vi "点位模式.vi"() -> ()   [LabVIEW 2020]
uses:
  VIs/gts.lvlib
  VI1s/gts1.lvlib
panel:
  in  "Tab Control":enum32{"Page 1", "Page 2"}(tab)
  in  "Jog运动":bool
  in  "pPrm 3":cluster{"acc":dbl, "dec":dbl, "smooth":dbl}={"acc"=1.0, "dec"=1.0, "smooth"=0.0}
  out "PrfJog return":i16
  in  "vel 2":dbl=30.0
  out "setPrm return":i16
  out "setVel return":i16
  out "Update return":i16
  out "clrsts return":i16
  in  "清除状态":bool
  out "stage 3":i16
  out "comparestop return":i16[](array[numeric])
  out "比较2return":i16[](array[numeric])
  out "比较1return":i16[](array[numeric])
  out "comparestart return":i16[](array[numeric])
  in  "pPrm 4":T1={"encx"=1, "ency"=2, "source"=0, "outputType"=0, "startLevel"=1, "time"=20000, "maxerr"=20, "threshold"=0}
  out "布尔数组":bool[](array[boolean])
  out "pSts 2":i32
  out "error":i16
  out "pStatus out":i16
  out "pValue out 2":i32
  out "function return 7":i16
  out "function return 6":i16
  in  "pBuf1":i32[](array[numeric])
  in  "一维位置比较":bool
  out "添加的数组":i16[](array[numeric])
  in  "pCrdPrm 2":T2={"dimension"=3, "profile[0]"=1, "profile[1]"=2, "profile[2]"=3, "profile[3]"=0, "profile[4]"=0, "profile[5]"=0, "profile[6]"=0, "profile[7]"=0, "@dummy control@"=0, "@dummy control@"=0, "@dummy control@"=0, "@dummy control@"=0, "@dummy control@"=0, "@dummy control@"=0, "synVelMax"=10.0, "synAccMax"=1.0, "evenTime"=10, "setOriginFlag"=0, "originPos[0]"=0, "originPos[1]"=0, "originPos[2]"=0, "originPos[3]"=0, "originPos[4]"=0, "originPos[5]"=0, "originPos[6]"=0, "originPos[7]"=0}
  in  "三轴直线插补":bool
  out "x = y?":bool
  out "stage 2":i16
  out "stage":i16
  out "close return":i16
  in  "关卡":bool
  in  "启动位置比较":bool
  in  "停止位置比较":bool
  in  "pBuf":cluster{"px":i32, "py":i32}[](array[cluster])=[{"px"=0, "py"=5000}, {"px"=0, "py"=8000}, {"px"=0, "py"=10000}, {"px"=0, "py"=15000}, {"px"=0, "py"=18000}, {"px"=0, "py"=20000}]
  in  "pPrm 2":T1={"encx"=1, "ency"=1, "source"=0, "outputType"=0, "startLevel"=1, "time"=20000, "maxerr"=20, "threshold"=0}
  in  "位置比较":bool
  in  "mdl":i16
  out "function return 3":i16
  in  "value":u16
  in  "index":i16
  in  "SetDo":bool
  out "function return 2":i16
  in  "路径 2":path
  out "function return":i16
  in  "pDllName":string
  in  "初始化扩展模块":bool
  out "homezero return 3":i16
  out "gohome return 3":i16
  out "get home prm return 3":i16
  in  "插补10000段":bool
  out "pSpace out":i32
  out "捕获次数":i32
  out "pValue out":i32
  out "追踪次数":i32
  in  "自动测试":bool
  in  "pEvent":T3={"loop"=1, "type"=30000, "index"=1, "id"=1, "condition"=3, "@dummy control@"=0, "@dummy control@"=0, "@dummy control@"=0, "@dummy control@"=0, "value"=50000.0}
  in  "pTaskData":cluster{"mask":i16, "option":i16}={"mask"=1, "option"=0}
  in  "主轴":i16=1
  in  "从轴":i16=2
  in  "单次测试":bool
  out "捕获数组":i32[](array[numeric])
  in  "打开home捕获":bool
  in  "pLookAheadBuf":T4(array[cluster])
  in  "数据路径":path=path "C:/Users/Admin/Desktop/固高资料/watch/Crd_data.txt"
  in  "轴号":T5(ring)=enum."2"
  out "闭环返回值":i16[](array[numeric])
  in  "闭环PID参数":T6={"kp"=2.0, "ki"=0.0, "kd"=0.0, "kvff"=0.0, "kaff"=0.0, "integralLimit"=0, "derivativeLimit"=0, "limit"=32767}
  in  "闭环控制":bool
  out "updatemotion return":i16
  in  "更新运动":bool
  out "zero return":i16
  in  "清零":bool
  out "CrdStart return":i16
  out "crddata return":i16
  out "Lnxy return":i16
  out "setCrd return":i16
  out "lookahead":i16
  in  "pCrdPrm":T2={"dimension"=2, "profile[0]"=1, "profile[1]"=2, "profile[2]"=0, "profile[3]"=0, "profile[4]"=0, "profile[5]"=0, "profile[6]"=0, "profile[7]"=0, "@dummy control@"=0, "@dummy control@"=0, "@dummy control@"=0, "@dummy control@"=0, "@dummy control@"=0, "@dummy control@"=0, "synVelMax"=10.0, "synAccMax"=1.0, "evenTime"=10, "setOriginFlag"=0, "originPos[0]"=0, "originPos[1]"=0, "originPos[2]"=0, "originPos[3]"=0, "originPos[4]"=0, "originPos[5]"=0, "originPos[6]"=0, "originPos[7]"=0}
  in  "前瞻":bool
  in  "插补运动":bool
  out "实际速度":dbl[](array[numeric])=[0.0, 0.0, 0.0, 0.0, 0.0, 0.0, 0.0, 1.0]
  out "encvel return":i16=-5
  out "实际位置":dbl[](array[numeric])=[0.0, 0.0, 0.0, 0.0, 0.0, 0.0, 0.0, 1.0]
  out "encpos return":i16=-5
  out "规划位置":dbl[](array[numeric])=[0.0, 0.0, 0.0, 0.0, 0.0, 0.0, 0.0, 1.0]
  out "prfpos return":i16=-5
  out "规划速度":dbl[](array[numeric])=[0.0, 0.0, 0.0, 0.0, 0.0, 0.0, 0.0, 1.0]
  out "prfvel return":i16=-5
  out "homezero return":i16
  out "gethomests return":i16
  out "pHomeStatus out":T7={"run"=0, "stage"=100, "error"=0, "pad1"=0, "capturePos"=-1, "targetPos"=-1}
  out "gohome return":i16
  out "get home prm return":i16
  in  "pHomePrm":T8={"mode"=11, "moveDir"=1, "indexDir"=1, "edge"=0, "triggerIndex"=-1, "pad1[0]"=0, "pad1[1]"=0, "pad1[2]"=0, "velHigh"=100.0, "velLow"=3.0, "acc"=1.0, "dec"=1.0, "smoothTime"=20, "pad2[0]"=0, "pad2[1]"=1, "pad2[2]"=0, "homeOffset"=0, "searchHomeDistance"=0, "searchIndexDistance"=0, "escapeStep"=2000, "pad3[0]"=0, "pad3[1]"=0}
  out "JogStop return":i16
  out "getPrm return":i16
  in  "回原点":bool
  out "reset return":i16
  out "Axisoff return":i16
  out "stopreturn":i16
  out "updatereturn":i16
  out "pos return":i16
  out "vel return":i16
  in  "vel":dbl=30.0
  in  "pos":i32=50000
  out "set prmreturn":i16
  out "get prm return":i16
  in  "pPrm":T9={"acc"=1.0, "dec"=1.0, "velStart"=0.0, "smoothTime"=20}
  out "set trap return":i16
  out "Axison return":i16
  out "clrsts return":i16
  out "config return":i16
  in  "路径":path=path "C:/Users/Admin/Desktop/GTS800.cfg"
  out "open return":i16
  in  "关伺服":bool
  in  "停止":bool
  in  "点位运动":bool
  in  "开伺服":bool
  in  "开卡":bool
  # "位置速度显示"
  # "函数返回值"
  # "点位运动参数"
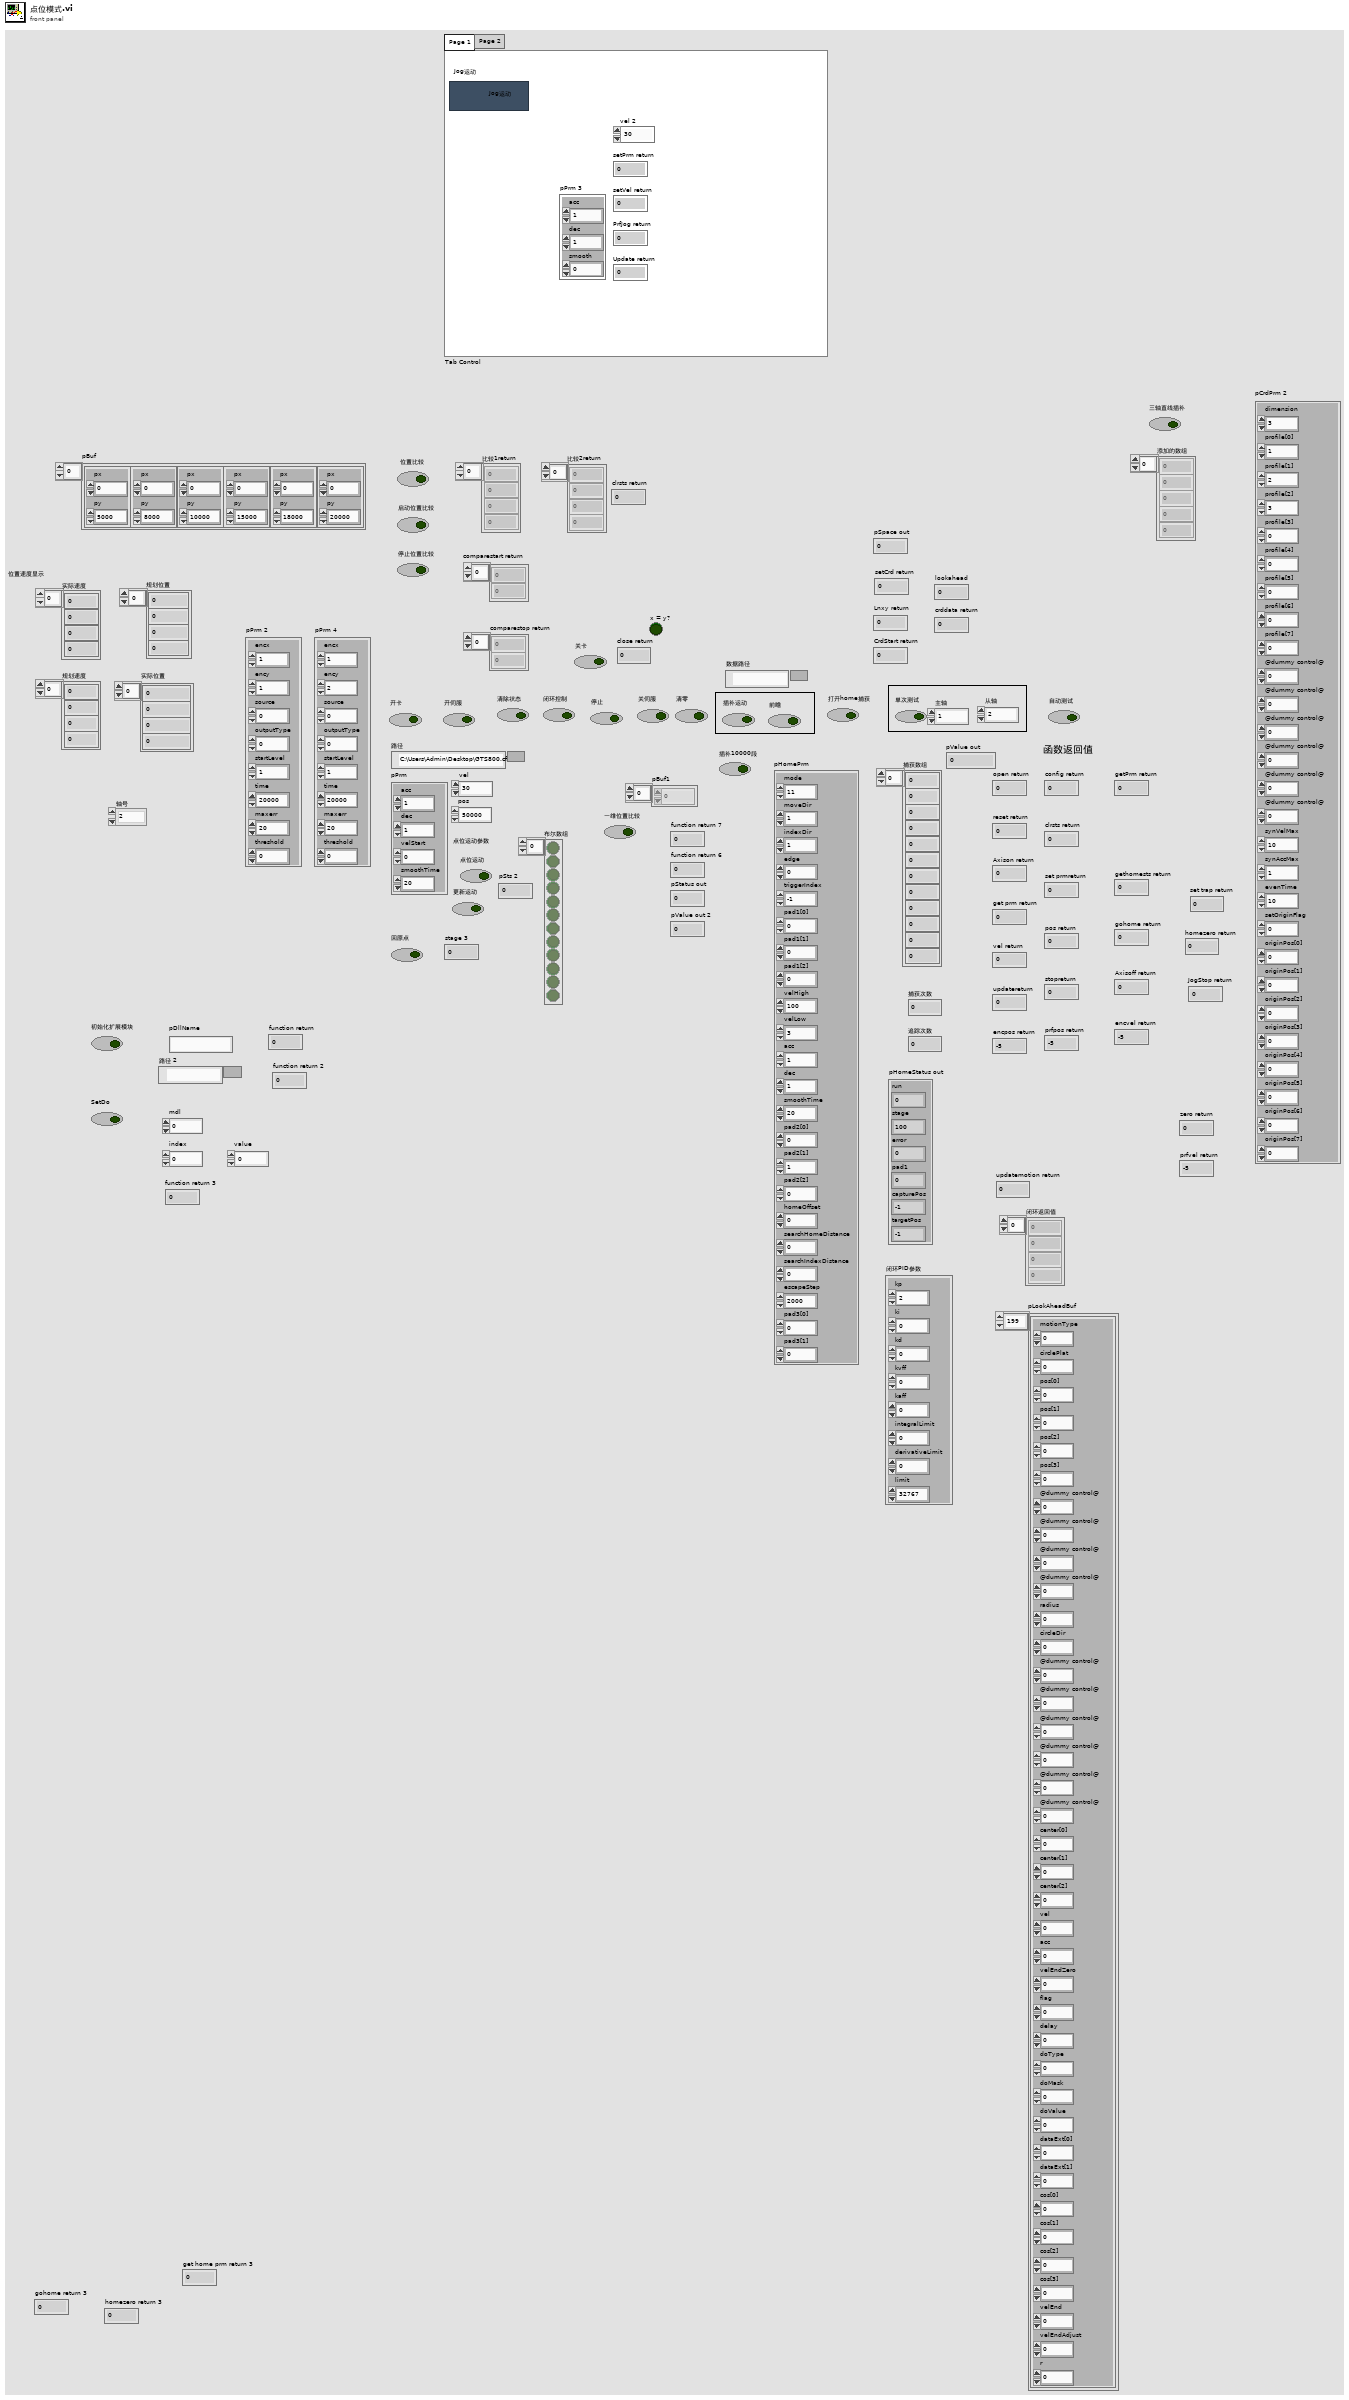
[diagram p1: front panel]
types:
  T1 = cluster{"encx":i16, "ency":i16, "source":i16, "outputType":i16, "startLevel":i16, "time":i16, "maxerr":i16, "threshold":i16}
  T2 = cluster{"dimension":i16, "profile[0]":i16, "profile[1]":i16, "profile[2]":i16, "profile[3]":i16, "profile[4]":i16, "profile[5]":i16, "profile[6]":i16, "profile[7]":i16, "@dummy control@":i8, "@dummy control@":i8, "@dummy control@":i8, "@dummy control@":i8, "@dummy control@":i8, "@dummy control@":i8, "synVelMax":dbl, "synAccMax":dbl, "evenTime":i16, "setOriginFlag":i16, "originPos[0]":i32, "originPos[1]":i32, "originPos[2]":i32, "originPos[3]":i32, "originPos[4]":i32, "originPos[5]":i32, "originPos[6]":i32, "originPos[7]":i32}
  T3 = cluster{"loop":u32, "type":u16, "index":u16, "id":u16, "condition":u16, "@dummy control@":i8, "@dummy control@":i8, "@dummy control@":i8, "@dummy control@":i8, "value":dbl}
  T4 = cluster{"motionType":i16, "circlePlat":i16, "pos[0]":i32, "pos[1]":i32, "pos[2]":i32, "pos[3]":i32, "@dummy control@":i8, "@dummy control@":i8, "@dummy control@":i8, "@dummy control@":i8, "radius":dbl, "circleDir":i16, "@dummy control@":i8, "@dummy control@":i8, "@dummy control@":i8, "@dummy control@":i8, "@dummy control@":i8, "@dummy control@":i8, "center[0]":dbl, "center[1]":dbl, "center[2]":dbl, "vel":dbl, "acc":dbl, "velEndZero":i16, "flag":i16, "delay":u16, "doType":i16, "doMask":u16, "doValue":u16, "dataExt[0]":u16, "dataExt[1]":u16, "cos[0]":dbl, "cos[1]":dbl, "cos[2]":dbl, "cos[3]":dbl, "velEnd":dbl, "velEndAdjust":dbl, "r":dbl}[]
  T5 = enum16{"none", "1", "2", "3", "4", "5", "6", "7", "8"}
  T6 = cluster{"kp":dbl, "ki":dbl, "kd":dbl, "kvff":dbl, "kaff":dbl, "integralLimit":i32, "derivativeLimit":i32, "limit":i16}
  T7 = cluster{"run":i16, "stage":i16, "error":i16, "pad1":i16, "capturePos":i32, "targetPos":i32}
  T8 = cluster{"mode":i16, "moveDir":i16, "indexDir":i16, "edge":i16, "triggerIndex":i16, "pad1[0]":i16, "pad1[1]":i16, "pad1[2]":i16, "velHigh":dbl, "velLow":dbl, "acc":dbl, "dec":dbl, "smoothTime":i16, "pad2[0]":i16, "pad2[1]":i16, "pad2[2]":i16, "homeOffset":i32, "searchHomeDistance":i32, "searchIndexDistance":i32, "escapeStep":i32, "pad3[0]":i32, "pad3[1]":i32}
  T9 = cluster{"acc":dbl, "dec":dbl, "velStart":dbl, "smoothTime":i16}
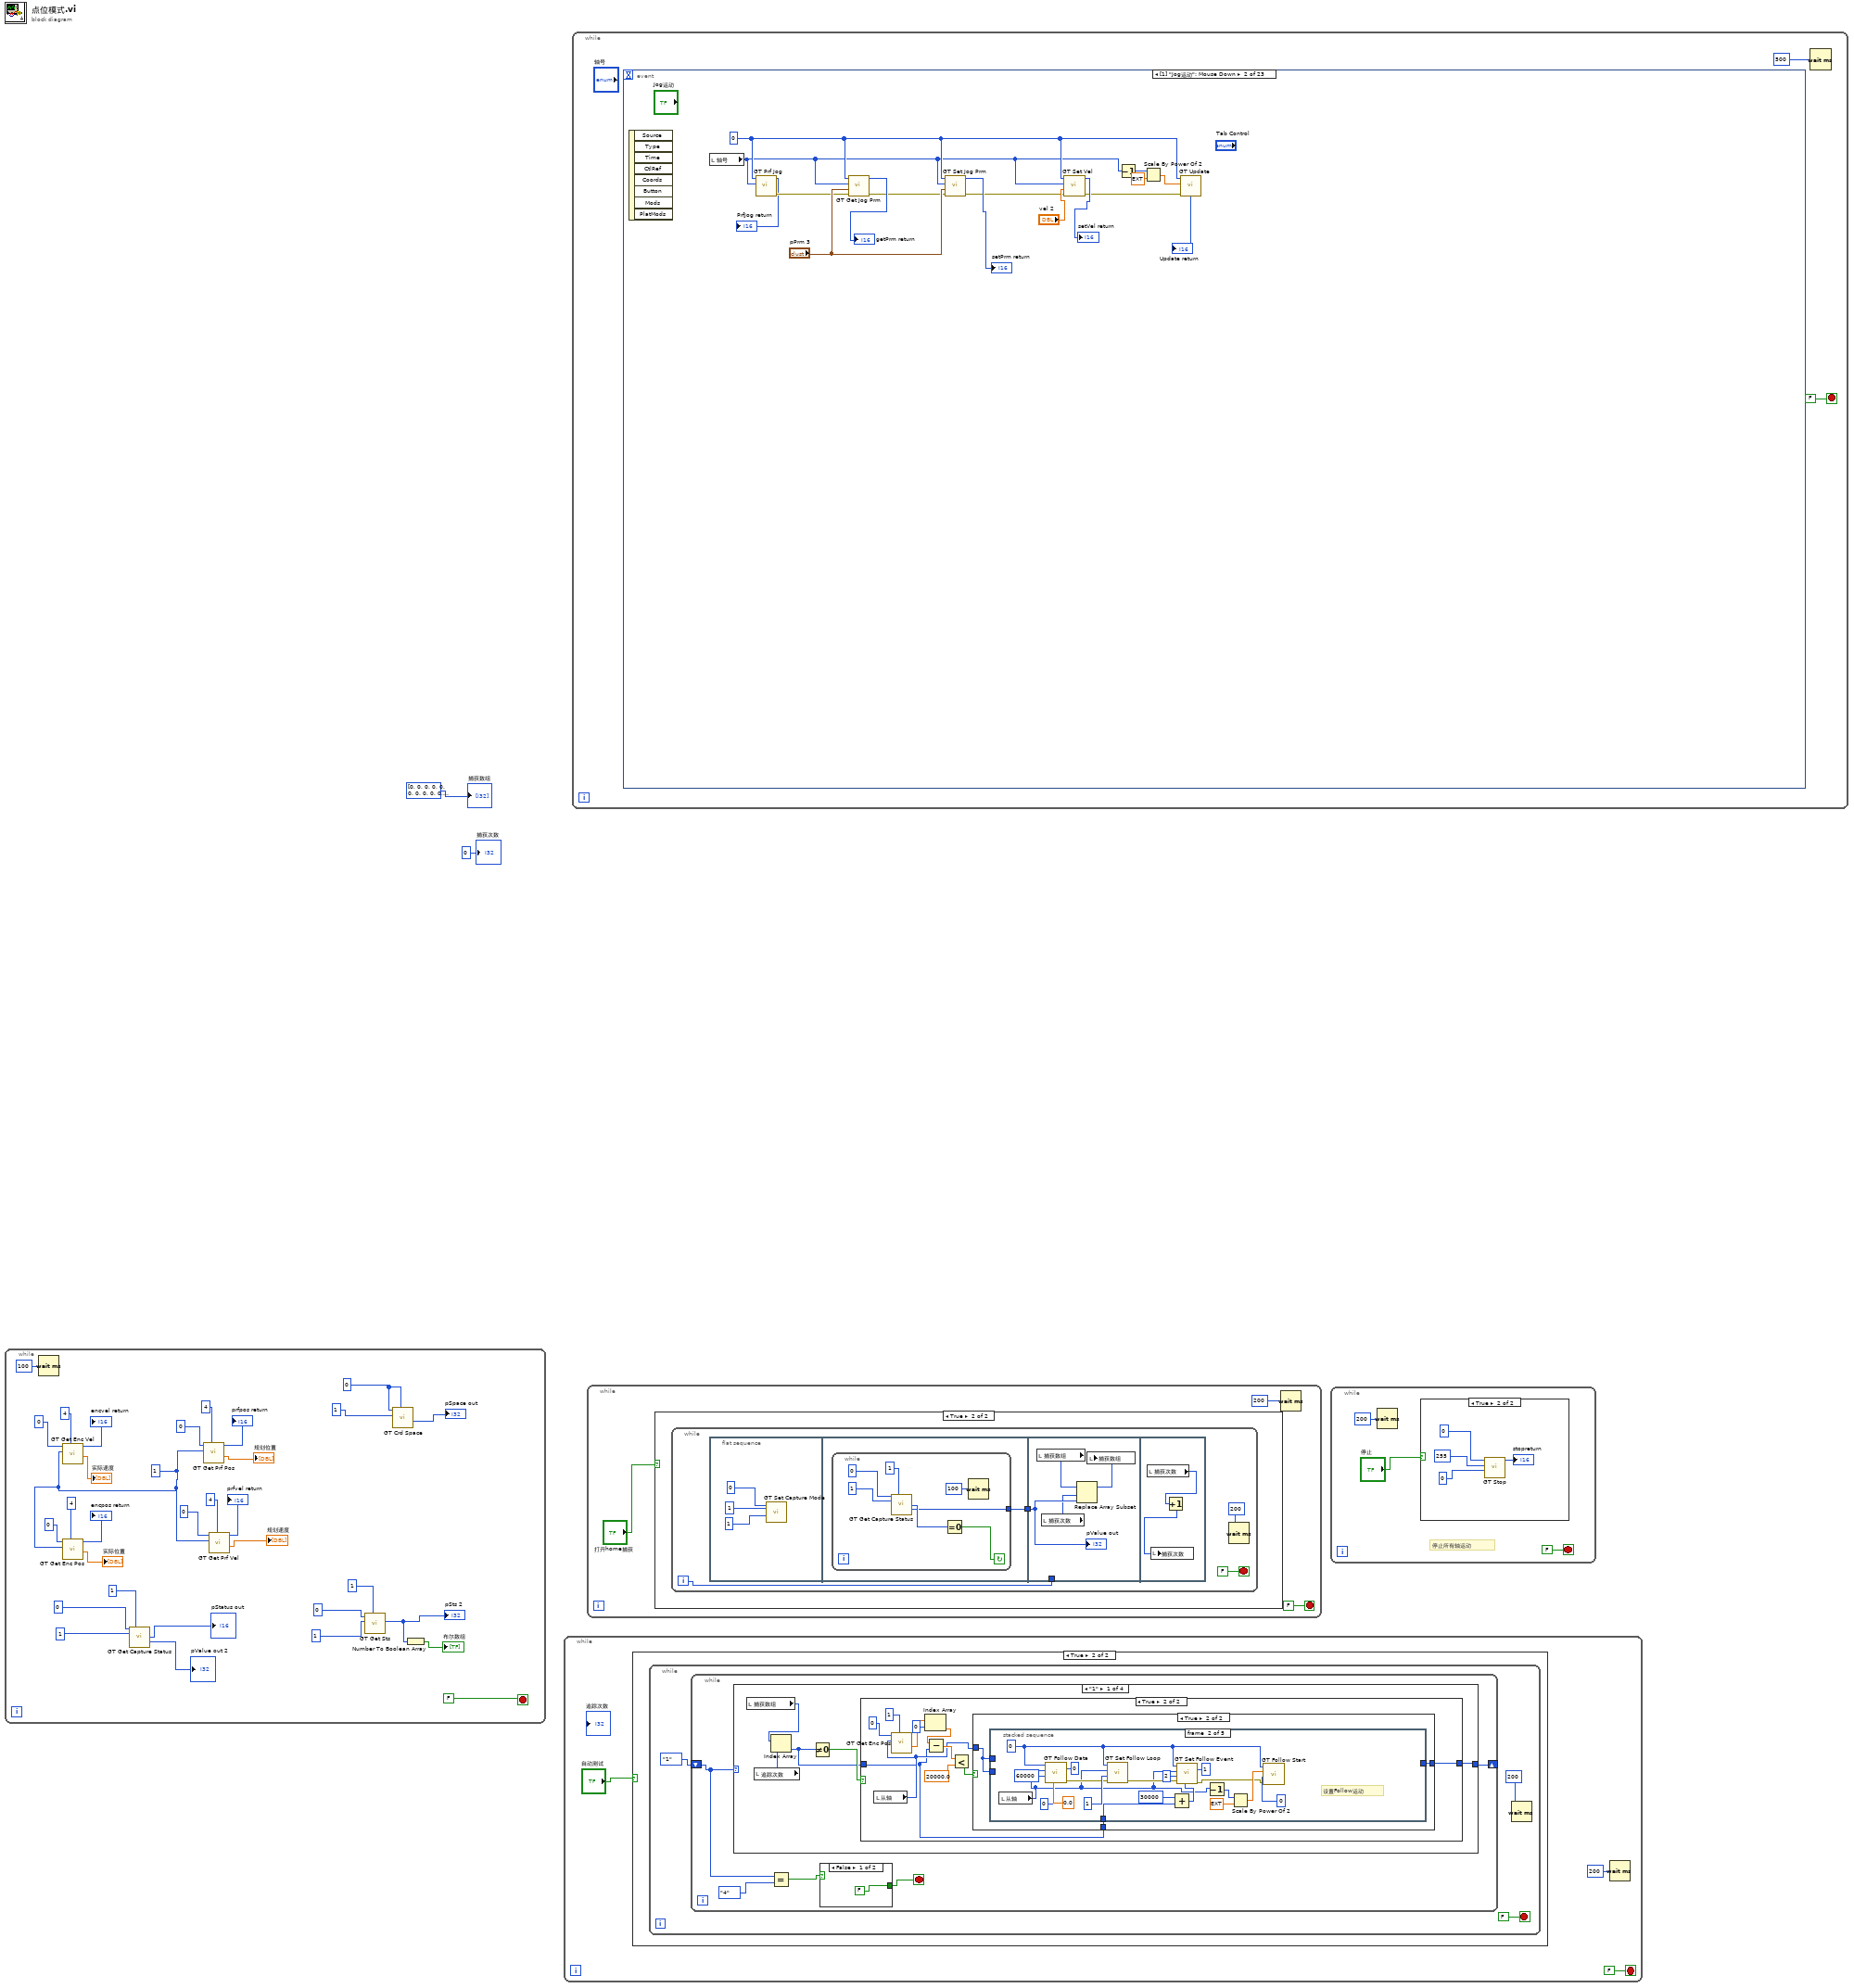
[diagram p0: block diagram]
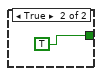
[diagram p3: hidden frame]
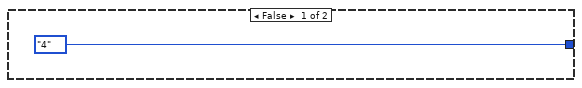
[diagram p4: hidden frame]
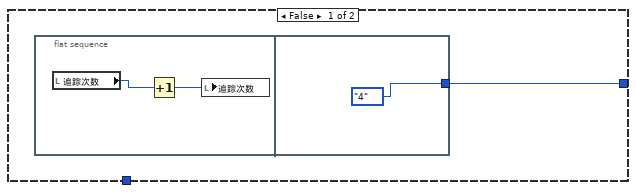
[diagram p5: hidden frame]
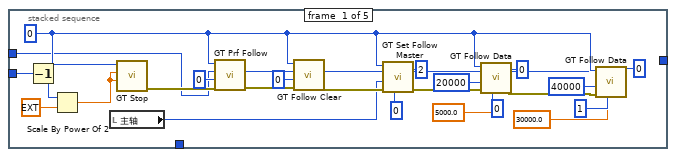
[diagram p6: hidden frame]
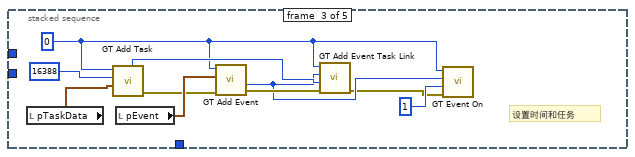
[diagram p7: hidden frame]
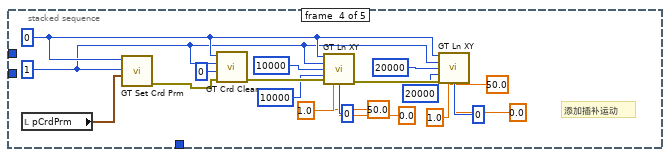
[diagram p8: hidden frame]
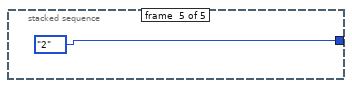
[diagram p9: hidden frame]
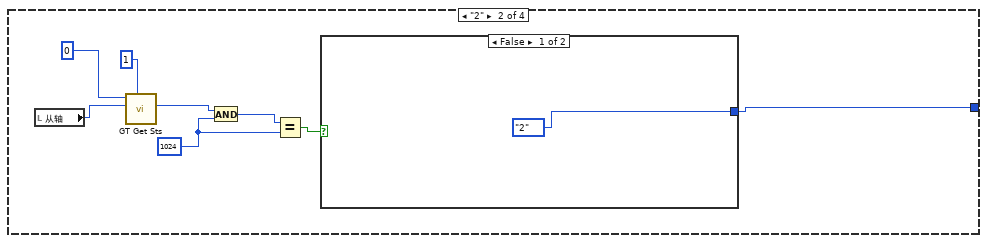
[diagram p10: hidden frame]
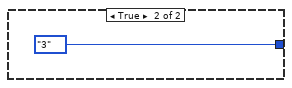
[diagram p11: hidden frame]
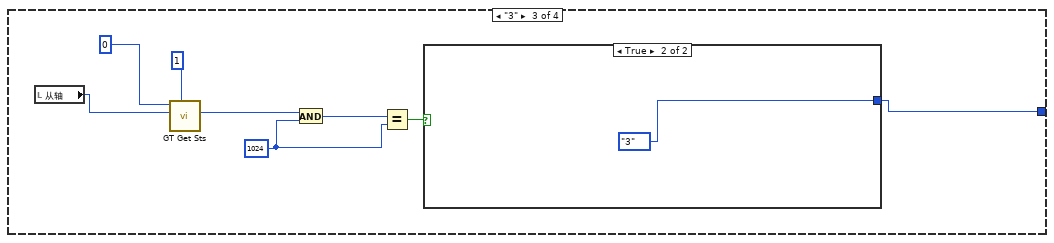
[diagram p12: hidden frame]
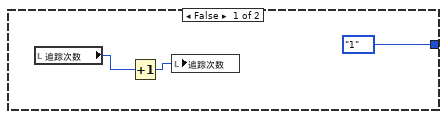
[diagram p13: hidden frame]
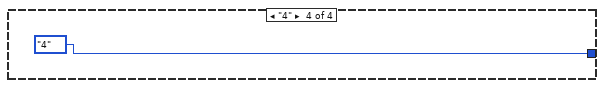
[diagram p14: hidden frame]
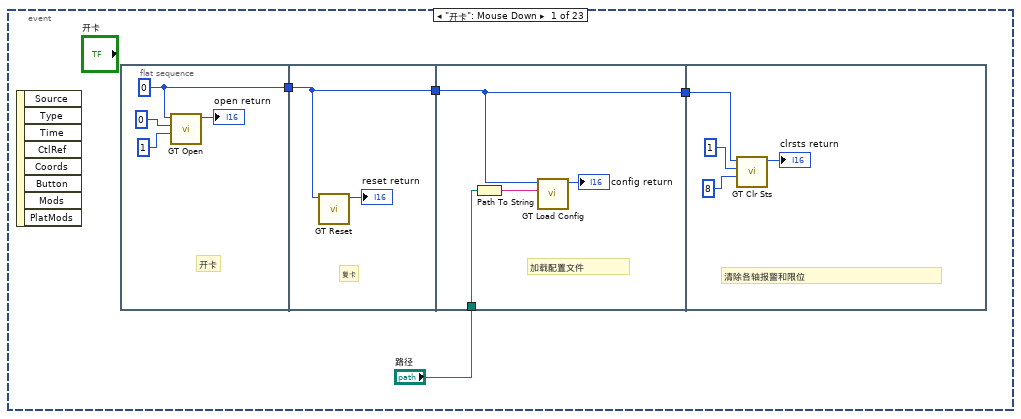
[diagram p17: hidden frame]
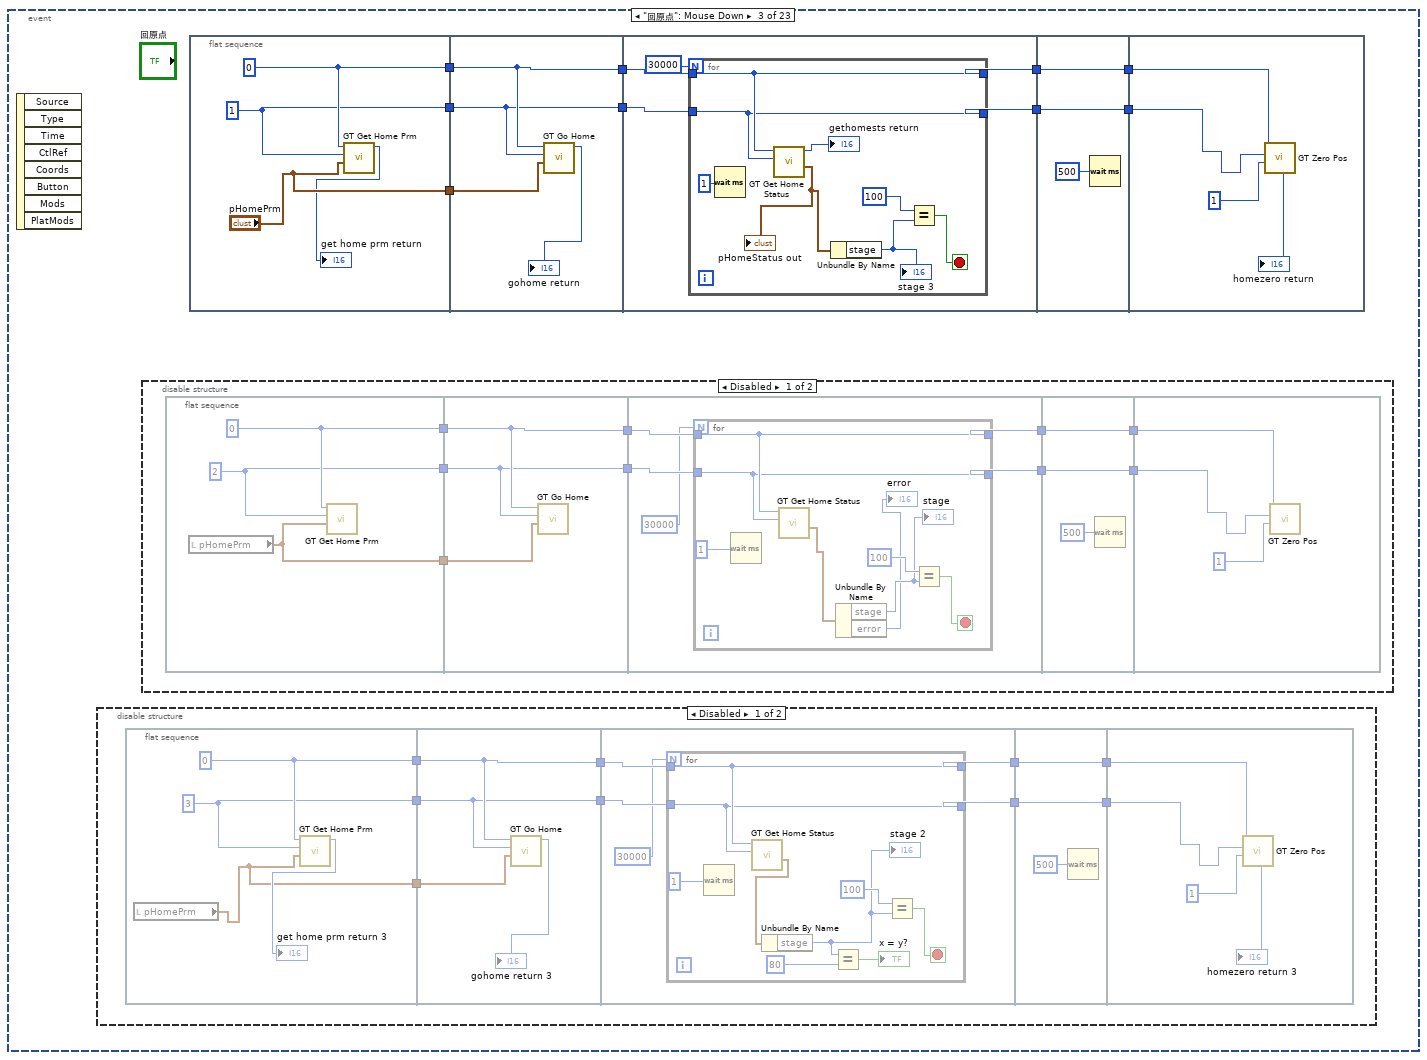
[diagram p18: hidden frame]
diagram:
  n1 = while {
    stop <- FALSE stop-if-true
    w14 = 0
    w16 = i16 1 ("profile")
    n2 = Wait (ms)(milliseconds to wait=u32 100 ("等待时间（毫秒）")) -> ()  [unwired: 1 out]
    n3 = call "GT Get Enc Vel.vi"("count"=i16 4, "encoder"=w16, "cardNum"=i16 0 ("encoder")) -> ("pValue out"=→"实际速度":dbl[], "function return"=→"encvel return":i16)  [unwired: 5 in, 2 out]
    n4 = call "GT Get Enc Pos.vi"("count"=i16 4, "encoder"=w16, "cardNum"=i16 0 ("encoder")) -> ("pValue out"=→"实际位置":dbl[], "function return"=→"encpos return":i16)  [unwired: 5 in, 2 out]
    n5 = call "GT Get Capture Status.vi"("cardNum"=0, "count"=1, "encoder"=1) -> ("pStatus out"=→"pStatus out":i16, "pValue out"=→"pValue out 2":i32)  [unwired: 8 in, 3 out]
    n6 = call "GT Get Prf Pos.vi"("count"=i16 4, "profile"=w16, "cardNum"=i16 0 ("profile")) -> ("pValue out"=→"规划位置":dbl[], "function return"=→"prfpos return":i16)  [unwired: 5 in, 2 out]
    n7 = call "GT Get Prf Vel.vi"("count"=i16 4, "profile"=w16, "cardNum"=i16 0 ("profile")) -> ("pValue out"=→"规划速度":dbl[], "function return"=→"prfvel return":i16)  [unwired: 5 in, 2 out]
    n8 = call "GT Get Sts.vi"("count"=1, "axis"=1, "cardNum"=0) -> ("pSts 2"=w4:i32)  [unwired: 5 in, 3 out]
    "pSts 2" <- w4
    n9 = call "GT Crd Space.vi"("fifo"=w14, "crd"=1, "cardNum"=w14) -> ("pSpace out"=→"pSpace out":i32)  [unwired: 6 in, 2 out]
    n10 = Number To Boolean Array(number=w4) -> (Boolean array=→"布尔数组":bool[])
  }
  n11 = while {
    stop <- FALSE stop-if-true
    n12 = case shown="True" "自动测试" {
      frame False {
      }
      frame True {
        n13 = while {
          stop <- FALSE stop-if-true
          n14 = while {
            shift-right: [w45] -> _
            shift-left: enum16{"1", "2", "3", "4"}."1" -> [w44]
            stop <- w41 stop-if-true
            n15 = case shown="\"1\"" w44 {
              tunnel: [w49 w145 w155 enum16{"1", "2", "3", "4"}."4"] -> w45
              frame "1" {
                n16 = local read "捕获数组"() -> (w52:i32[])
                n17 = local read "追踪次数"() -> (w51:i32)
                n18 = Index Array(array=w52, index=w51) -> (element=w48:i32)
                n19 = Not Equal To 0?(x=w48) -> (x != 0?=w50:bool)
                n20 = case shown="True" w50 {
                  tunnel: [enum16{"1", "2", "3", "4"}."4" w54] -> w49
                  tunnel: w48 -> [_ w55]
                  frame False {
                  }
                  frame True {
                    n21 = local read "从轴"() -> (w56:i16)
                    n22 = call "GT Get Enc Pos.vi"("count"=i16 1, "encoder"=w56, "cardNum"=i16 0) -> ("pValue out"=w61:dbl[])  [unwired: 5 in, 3 out]
                    n23 = Index Array(array=w61, index=0 ("索引")) -> (element=w59:dbl)
                    n24 = Subtract(x=w59, y=w55) -> (x-y=w62:dbl)
                    n25 = Less?(x=w62, y=20000.0) -> (x < y?=w57:bool)
                    n26 = case shown="True" w57 {
                      tunnel: w56 -> [_ w71]
                      tunnel: w55 -> [_ w70]
                      tunnel: [w65 w69] -> w54
                      frame False {
                        n27 = flat-sequence {
                          tunnel: [enum16{"1", "2", "3", "4"}."4"] -> w65
                          frame #0 {
                            n28 = local read "追踪次数"() -> (w67:i32)
                            n29 = Increment(x=w67) -> (x+1=w66:i32)
                            n30 = local write "追踪次数"(w66) -> ()
                          }
                          frame #1 {
                          }
                        }
                      }
                      frame True {
                        n31 = stacked-sequence {
                          tunnel: w71 -> [w94 _ _ _ _]
                          tunnel: w71 -> [w77 _ _ _ _]
                          tunnel: w70 -> [_ w105 _ _ _]
                          tunnel: [_ _ _ _ enum16{"1", "2", "3", "4"}."2"] -> w69
                          frame #0 {
                            w78 = i16 0 ("cardNum")
                            n32 = Decrement(x=w94) -> (x-1=w95:i16)
                            n33 = Scale By Power Of 2(n=w95, x=ext 1.0) -> (x*2^n=w92:ext)
                            n34 = local read "主轴"() -> (w86:i16)
                            n35 = call "GT Stop.vi"("option"=w92, "mask"=w92, "cardNum"=w78) -> ("error out"=w91:errorcluster)  [unwired: 7 in, 1 out]
                            n36 = call "GT Prf Follow.vi"("error in (no error)"=w91, "dir"=i16 0, "profile"=w77, "cardNum"=w78) -> ("error out"=w89:errorcluster)  [unwired: 6 in, 1 out]
                            n37 = call "GT Follow Clear.vi"("error in (no error)"=w89, "fifo"=i16 0, "profile"=w77, "cardNum"=w78) -> ("error out"=w87:errorcluster)  [unwired: 6 in, 1 out]
                            n38 = call "GT Set Follow Master.vi"("masterItem"=i16 0, "masterType"=i16 2, "error in (no error)"=w87, "masterIndex"=w86, "profile"=w77, "cardNum"=w78) -> ("error out"=w83:errorcluster)  [unwired: 4 in, 1 out]
                            n39 = call "GT Follow Data.vi"("fifo"=i16 0, "type"=i16 0, "slaveSegment"=5000.0, "error in (no error)"=w83, "masterSegment"=20000, "profile"=w77, "cardNum"=w78) -> ("error out"=w74:errorcluster)  [unwired: 3 in, 1 out]
                            n40 = call "GT Follow Data.vi"("fifo"=i16 0, "type"=i16 1, "slaveSegment"=30000.0, "error in (no error)"=w74, "masterSegment"=40000, "profile"=w77, "cardNum"=w78) -> ()  [unwired: 3 in, 2 out]
                          }
                          frame #1 {
                            w102 = i16 0 ("cardNum")
                            # "设置Follow运动"
                            n41 = local read "从轴"() -> (w98:i16)
                            n42 = call "GT Follow Data.vi"("fifo"=i16 0, "type"=i16 0, "slaveSegment"=0.0, "masterSegment"=60000, "profile"=w98, "cardNum"=w102) -> ("error out"=w109:errorcluster)  [unwired: 4 in, 1 out]
                            n43 = call "GT Set Follow Loop.vi"("error in (no error)"=w109, "loop"=1, "profile"=w98, "cardNum"=w102) -> ("error out"=w108:errorcluster)  [unwired: 6 in, 1 out]
                            n44 = Add(x=30000, y=w105) -> (x+y=w103:i32)
                            n45 = call "GT Set Follow Event.vi"("pos"=w103, "masterDir"=i16 1, "error in (no error)"=w108, "event"=i16 2, "profile"=w98, "cardNum"=w102) -> ("error out"=w96:errorcluster)  [unwired: 4 in, 1 out]
                            n46 = Decrement(x=w98) -> (x-1=w100:i16)
                            n47 = Scale By Power Of 2(n=w100, x=ext 1.0) -> (x*2^n=w97:ext)
                            n48 = call "GT Follow Start.vi"("error in (no error)"=w96, "option"=0, "mask"=w97, "cardNum"=w102) -> ()  [unwired: 6 in, 2 out]
                          }
                          frame #2 {
                            w118 = i16 0 ("cardNum")
                            # "设置时间和任务"
                            n49 = local read "pTaskData"() -> (w123:cluster{"mask":i16, "option":i16})
                            n50 = call "GT Add Task.vi"("pTaskData"=w123, "taskType"=i16 16388, "cardNum"=w118) -> ("error out"=w121:errorcluster, "pTaskIndex out"=w119:i16)  [unwired: 5 in, 2 out]
                            n51 = local read "pEvent"() -> (w122:T3)
                            n52 = call "GT Add Event.vi"("error in (no error)"=w121, "pEvent"=w122, "cardNum"=w118) -> ("error out"=w120:errorcluster, "pEventIndex out"=w117:i16)  [unwired: 5 in, 2 out]
                            n53 = call "GT Add Event Task Link.vi"("error in (no error)"=w120, "taskIndex"=w119, "eventIndex"=w117, "cardNum"=w118) -> ("error out"=w115:errorcluster)  [unwired: 5 in, 2 out]
                            n54 = call "GT Event On.vi"("error in (no error)"=w115, "count"=i16 1, "eventIndex"=w117, "cardNum"=w118) -> ()  [unwired: 6 in, 2 out]
                          }
                          frame #3 {
                            w131 = i16 1 ("crd")
                            w132 = i16 0 ("cardNum")
                            # "添加插补运动"
                            n55 = local read "pCrdPrm"() -> (w143:T2)
                            n56 = call "GT Set Crd Prm.vi"("pCrdPrm"=w143, "crd"=w131, "cardNum"=w132) -> ("error out"=w141:errorcluster)  [unwired: 7 in, 1 out]
                            n57 = call "GT Crd Clear.vi"("error in (no error)"=w141, "fifo"=i16 0, "crd"=w131, "cardNum"=w132) -> ("error out"=w140:errorcluster)  [unwired: 6 in, 1 out]
                            n58 = call "GT Ln XY.vi"("cardNum"=w132, "synVel"=50.0, "velEnd"=0.0, "crd"=w131, "x"=10000, "y"=10000, "error in (no error)"=w140, "synAcc"=1.0, "fifo"=i16 0) -> ("error out"=w133:errorcluster)  [unwired: 5 in, 1 out]
                            n59 = call "GT Ln XY.vi"("cardNum"=w132, "synVel"=50.0, "velEnd"=0.0, "crd"=w131, "x"=20000, "y"=20000, "error in (no error)"=w133, "synAcc"=1.0, "fifo"=i16 0) -> ()  [unwired: 5 in, 2 out]
                          }
                          frame #4 {
                          }
                        }
                      }
                    }
                  }
                }
              }
              frame "2" {
                w148 = 1024 ("y")
                n60 = local read "从轴"() -> (w151:i16)
                n61 = call "GT Get Sts.vi"("count"=i16 1, "axis"=w151, "cardNum"=i16 0) -> ("pSts 2"=w149:i32)  [unwired: 5 in, 3 out]
                n62 = And(x=w149, y=w148) -> (x .and. y?=w147:i32)
                n63 = Equal?(x=w147, y=w148) -> (x = y?=w146:bool)
                n64 = case shown="False" w146 {
                  tunnel: [enum16{"1", "2", "3", "4"}."2" enum16{"1", "2", "3", "4"}."3"] -> w145
                  frame False {
                  }
                  frame True {
                  }
                }
              }
              frame "3" {
                w157 = 1024 ("y")
                n65 = local read "从轴"() -> (w161:i16)
                n66 = call "GT Get Sts.vi"("count"=i16 1, "axis"=w161, "cardNum"=i16 0) -> ("pSts 2"=w159:i32)  [unwired: 5 in, 3 out]
                n67 = And(x=w159, y=w157) -> (x .and. y?=w158:i32)
                n68 = Equal?(x=w158, y=w157) -> (x = y?=w156:bool)
                n69 = case shown="True" w156 {
                  tunnel: [enum16{"1", "2", "3", "4"}."1" enum16{"1", "2", "3", "4"}."3"] -> w155
                  frame False {
                    n70 = local read "追踪次数"() -> (w165:i32)
                    n71 = Increment(x=w165) -> (x+1=w164:i32)
                    n72 = local write "追踪次数"(w164) -> ()
                  }
                  frame True {
                  }
                }
              }
              frame "4" {
              }
            }
            n73 = Equal?(x=w44, y=enum16{"1", "2", "3", "4"}."4") -> (x = y?=w42:bool)
            n74 = case shown="False" w42 {
              tunnel: [FALSE TRUE] -> w41
              frame False {
              }
              frame True {
              }
            }
          }
          n75 = Wait (ms)(milliseconds to wait=u32 200 ("等待时间（毫秒）")) -> ()  [unwired: 1 out]
        }
      }
    }
    n76 = Wait (ms)(milliseconds to wait=u32 200 ("等待时间（毫秒）")) -> ()  [unwired: 1 out]
  }
  n77 = while {
    stop <- FALSE stop-if-true
    n78 = event shown="[1] \"Jog运动\": Mouse Down" {
      selector: _ -> [_ _ _ _ _ _ _ _ _ _ _ _ _ _ _ _ _ _ _ _ _ _ _]
      dyn-events: _ -> [_ _ _ _ _ _ _ _ _ _ _ _ _ _ _ _ _ _ _ _ _ _ _]
      timeout: _ -> [_ _ _ _ _ _ _ _ _ _ _ _ _ _ _ _ _ _ _ _ _ _ _]
      event "开卡": Mouse Down {
        n79 = event-data() -> ()  [unwired: 1 in, 8 out]
        n80 = flat-sequence {
          tunnel: [w176] -> w173
          tunnel: w173 -> [w178]
          tunnel: [w178] -> w172
          tunnel: w172 -> [w182]
          tunnel: [w182] -> w171
          tunnel: "路径" -> [w181]
          tunnel: w171 -> [w186]
          frame #0 {
            w176 = i16 0 ("channel")
            # "开卡"
            n81 = call "GT Open.vi"("param"=i16 1, "channel"=i16 0, "cardNum"=w176) -> ("function return"=→"open return":i16)  [unwired: 7 in, 1 out]
          }
          frame #1 {
            # "复卡"
            n82 = call "GT Reset.vi"("cardNum"=w178) -> ("function return"=→"reset return":i16)  [unwired: 9 in, 1 out]
          }
          frame #2 {
            # "加载配置文件"
            n83 = Path To String(path=w181) -> (string=w180:string)
            n84 = call "GT Load Config.vi"("pFile"=w180, "cardNum"=w182) -> ("function return"=→"config return":i16)  [unwired: 7 in, 2 out]
          }
          frame #3 {
            # "清除各轴报警和限位"
            n85 = call "GT Clr Sts.vi"("count"=i16 8, "axis"=i16 1, "cardNum"=w186) -> ("function return"=→"clrsts return":i16)  [unwired: 7 in, 1 out]
          }
        }
      }
      event "Jog运动": Mouse Down {
        w203 = i16 0 ("cardNum")
        n86 = event-data() -> ()  [unwired: 1 in, 8 out]
        n87 = local read "轴号"() -> (w190:T5)
        n88 = call "GT Prf Jog.vi"("profile"=w190, "cardNum"=w203) -> ("error out"=w201:errorcluster, "function return"=→"PrfJog return":i16)  [unwired: 8 in]
        n89 = call "GT Get Jog Prm.vi"("error in (no error)"=w201, "pPrm"="pPrm 3", "profile"=w190, "cardNum"=w203) -> ("error out"=w195:errorcluster, "function return"=→"getPrm return":i16)  [unwired: 5 in, 1 out]
        n90 = call "GT Set Jog Prm.vi"("error in (no error)"=w195, "pPrm"="pPrm 3", "profile"=w190, "cardNum"=w203) -> ("error out"=w194:errorcluster, "function return"=→"setPrm return":i16)  [unwired: 5 in, 1 out]
        n91 = call "GT Set Vel.vi"("error in (no error)"=w194, "vel"="vel 2", "profile"=w190, "cardNum"=w203) -> ("error out"=w193:errorcluster, "function return"=→"setVel return":i16)  [unwired: 6 in]
        n92 = Decrement(x=w190) -> (x-1=w192:T5)
        n93 = Scale By Power Of 2(n=w192, x=ext 1.0) -> (x*2^n=w189:ext)
        n94 = call "GT Update.vi"("error in (no error)"=w193, "mask"=w189, "cardNum"=w203) -> ("function return"=→"Update return":i16)  [unwired: 7 in, 1 out]
      }
      event "回原点": Mouse Down {
        n95 = event-data() -> ()  [unwired: 1 in, 8 out]
        n96 = disable-structure shown="Disabled" {
          frame Disabled {
            n97 = flat-sequence {
              tunnel: [w259] -> w255
              tunnel: [w256] -> w254
              tunnel: [w257] -> w253
              tunnel: w255 -> [w263]
              tunnel: [w263] -> w252
              tunnel: w254 -> [w262]
              tunnel: w253 -> [w260]
              tunnel: [w260] -> w251
              tunnel: w252 -> [w268]
              tunnel: [w267] -> w250
              tunnel: w251 -> [w266]
              tunnel: [w265] -> w249
              tunnel: w250 -> [w280]
              tunnel: [w280] -> w248
              tunnel: [w278] -> w247
              tunnel: w249 -> [w278]
              tunnel: w248 -> [w282]
              tunnel: w247 -> [w281]
              frame #0 {
                w257 = 3
                w259 = i16 0 ("cardNum")
                n98 = local read "pHomePrm"() -> (w256:T8)
                n99 = call "GT Get Home Prm.vi"("pHomePrm"=w256, "axis"=w257, "cardNum"=w259) -> ("function return"=→"get home prm return 3":i16)  [unwired: 6 in, 2 out]
              }
              frame #1 {
                n100 = call "GT Go Home.vi"("pHomePrm"=w262, "axis"=w260, "cardNum"=w263) -> ("function return"=→"gohome return 3":i16)  [unwired: 6 in, 2 out]
              }
              frame #2 {
                n101 = for {
                  N: 30000 -> [_]
                  tunnel: w268 -> [w276]
                  tunnel: [w276] -> w267
                  tunnel: w266 -> [w274]
                  tunnel: [w274] -> w265
                  stop <- w273 stop-if-true
                  n102 = Wait (ms)(milliseconds to wait=1) -> ()  [unwired: 1 out]
                  n103 = call "GT Get Home Status.vi"("axis"=w274, "cardNum"=w276) -> ("pHomeStatus out"=w275:T7)  [unwired: 7 in, 2 out]
                  n104 = Unbundle By Name(w275) -> ("stage"=w270:i16)
                  "stage 2" <- w270
                  n105 = Equal?(x=w270, y=80) -> (x = y?=→"x = y?":bool)
                  n106 = Equal?(x=i16 100, y=w270) -> (x = y?=w273:bool)
                }
              }
              frame #3 {
                n107 = Wait (ms)(milliseconds to wait=u32 500 ("等待时间（毫秒）")) -> ()  [unwired: 1 out]
              }
              frame #4 {
                n108 = call "GT Zero Pos.vi"("count"=i16 1, "axis"=w281, "cardNum"=w282) -> ("function return"=→"homezero return 3":i16)  [unwired: 7 in, 1 out]
              }
            }
          }
          frame Enabled {
          }
        }
        n109 = disable-structure shown="Disabled" {
          frame Disabled {
            n110 = flat-sequence {
              tunnel: [w224] -> w221
              tunnel: [w223] -> w220
              tunnel: [w222] -> w219
              tunnel: w221 -> [w227]
              tunnel: [w227] -> w218
              tunnel: w220 -> [w226]
              tunnel: [w226] -> w217
              tunnel: w219 -> [w225]
              tunnel: w218 -> [w232]
              tunnel: [w231] -> w216
              tunnel: w217 -> [w230]
              tunnel: [w229] -> w215
              tunnel: w216 -> [w243]
              tunnel: [w243] -> w214
              tunnel: [w241] -> w213
              tunnel: w215 -> [w241]
              tunnel: w214 -> [w245]
              tunnel: w213 -> [w244]
              frame #0 {
                w223 = 2
                w224 = i16 0 ("cardNum")
                n111 = local read "pHomePrm"() -> (w222:T8)
                n112 = call "GT Get Home Prm.vi"("pHomePrm"=w222, "axis"=w223, "cardNum"=w224) -> ()  [unwired: 6 in, 3 out]
              }
              frame #1 {
                n113 = call "GT Go Home.vi"("pHomePrm"=w225, "axis"=w226, "cardNum"=w227) -> ()  [unwired: 6 in, 3 out]
              }
              frame #2 {
                n114 = for {
                  N: 30000 -> [_]
                  tunnel: w232 -> [w239]
                  tunnel: [w239] -> w231
                  tunnel: w230 -> [w237]
                  tunnel: [w237] -> w229
                  stop <- w235 stop-if-true
                  n115 = Wait (ms)(milliseconds to wait=1) -> ()  [unwired: 1 out]
                  n116 = call "GT Get Home Status.vi"("axis"=w237, "cardNum"=w239) -> ("pHomeStatus out"=w238:T7)  [unwired: 7 in, 2 out]
                  n117 = Unbundle By Name(w238) -> ("stage"=w236:i16, "error"=→"error":i16)
                  "stage" <- w236
                  n118 = Equal?(x=i16 100, y=w236) -> (x = y?=w235:bool)
                }
              }
              frame #3 {
                n119 = Wait (ms)(milliseconds to wait=u32 500 ("等待时间（毫秒）")) -> ()  [unwired: 1 out]
              }
              frame #4 {
                n120 = call "GT Zero Pos.vi"("count"=i16 1, "axis"=w244, "cardNum"=w245) -> ()  [unwired: 7 in, 2 out]
              }
            }
          }
          frame Enabled {
          }
        }
        n121 = flat-sequence {
          tunnel: [w288] -> w212
          tunnel: ["pHomePrm"] -> w211
          tunnel: [w285] -> w210
          tunnel: w212 -> [w292]
          tunnel: [w292] -> w209
          tunnel: w211 -> [w291]
          tunnel: w210 -> [w289]
          tunnel: [w289] -> w208
          tunnel: w209 -> [w297]
          tunnel: [w296] -> w207
          tunnel: w208 -> [w295]
          tunnel: [w294] -> w206
          tunnel: w207 -> [w308]
          tunnel: [w308] -> w205
          tunnel: [w306] -> w204
          tunnel: w206 -> [w306]
          tunnel: w205 -> [w310]
          tunnel: w204 -> [w309]
          frame #0 {
            w285 = 1
            w288 = i16 0 ("cardNum")
            n122 = call "GT Get Home Prm.vi"("pHomePrm"="pHomePrm", "axis"=w285, "cardNum"=w288) -> ("function return"=→"get home prm return":i16)  [unwired: 6 in, 2 out]
          }
          frame #1 {
            n123 = call "GT Go Home.vi"("pHomePrm"=w291, "axis"=w289, "cardNum"=w292) -> ("function return"=→"gohome return":i16)  [unwired: 6 in, 2 out]
          }
          frame #2 {
            n124 = for {
              N: 30000 -> [_]
              tunnel: w297 -> [w304]
              tunnel: [w304] -> w296
              tunnel: w295 -> [w301]
              tunnel: [w301] -> w294
              stop <- w299 stop-if-true
              n125 = Wait (ms)(milliseconds to wait=1) -> ()  [unwired: 1 out]
              n126 = call "GT Get Home Status.vi"("axis"=w301, "cardNum"=w304) -> ("pHomeStatus out"=w302:T7, "function return"=→"gethomests return":i16)  [unwired: 7 in, 1 out]
              "pHomeStatus out" <- w302
              n127 = Unbundle By Name(w302) -> ("stage"=w300:i16)
              "stage 3" <- w300
              n128 = Equal?(x=i16 100, y=w300) -> (x = y?=w299:bool)
            }
          }
          frame #3 {
            n129 = Wait (ms)(milliseconds to wait=u32 500 ("等待时间（毫秒）")) -> ()  [unwired: 1 out]
          }
          frame #4 {
            n130 = call "GT Zero Pos.vi"("count"=i16 1, "axis"=w309, "cardNum"=w310) -> ("function return"=→"homezero return":i16)  [unwired: 7 in, 1 out]
          }
        }
      }
      event "Jog运动": Mouse Up {
        n131 = event-data() -> ()  [unwired: 1 in, 8 out]
        n132 = local read "轴号"() -> (w316:T5)
        n133 = Decrement(x=w316) -> (x-1=w315:T5)
        n134 = Scale By Power Of 2(n=w315, x=ext 1.0) -> (x*2^n=w313:ext)
        n135 = call "GT Stop.vi"("option"=0, "mask"=w313, "cardNum"=0 ("mask")) -> ("function return"=→"JogStop return":i16)  [unwired: 7 in, 1 out]
      }
      event "开伺服": Mouse Down {
        w321 = i16 0 ("axis")
        n136 = event-data() -> ()  [unwired: 1 in, 8 out]
        n137 = call "GT Axis On.vi"("axis"=i16 1, "cardNum"=w321) -> ("error out"=w324:errorcluster)  [unwired: 8 in, 1 out]
        n138 = call "GT Axis On.vi"("error in (no error)"=w324, "axis"=i16 2, "cardNum"=w321) -> ("function return"=→"Axison return":i16)  [unwired: 7 in, 1 out]
        n139 = call "GT Axis On.vi"("axis"=3, "cardNum"=w321) -> ()  [unwired: 8 in, 2 out]
        n140 = call "GT Axis On.vi"("axis"=4, "cardNum"=w321) -> ()  [unwired: 8 in, 2 out]
      }
      event "清除状态": Mouse Down {
        n141 = event-data() -> ()  [unwired: 1 in, 8 out]
        n142 = call "GT Clr Sts.vi"("count"=8, "axis"=1, "cardNum"=0) -> ("function return"=→"clrsts return":i16)  [unwired: 7 in, 1 out]
      }
      event "点位运动": Mouse Down {
        w337 = i16 0 ("cardNum")
        # "启动点位"
        # "设置目标位置和速度"
        # "设置点位参数"
        # "读取点位参数"
        # "设置点位模式"
        n143 = event-data() -> ()  [unwired: 1 in, 8 out]
        n144 = local read "轴号"() -> (w333:T5)
        n145 = call "GT Prf Trap.vi"("profile"=w333, "cardNum"=w337) -> ("error out"=w340:errorcluster, "function return"=→"set trap return":i16)  [unwired: 8 in]
        n146 = call "GT Get Trap Prm.vi"("error in (no error)"=w340, "pPrm"="pPrm", "profile"=w333, "cardNum"=w337) -> ("error out"=w339:errorcluster, "function return"=→"get prm return":i16)  [unwired: 5 in, 1 out]
        n147 = call "GT Set Trap Prm.vi"("error in (no error)"=w339, "pPrm"="pPrm", "profile"=w333, "cardNum"=w337) -> ("error out"=w338:errorcluster, "function return"=→"set prmreturn":i16)  [unwired: 5 in, 1 out]
        n148 = call "GT Set Pos.vi"("error in (no error)"=w338, "pos"="pos", "profile"=w333, "cardNum"=w337) -> ("error out"=w336:errorcluster, "function return"=→"pos return":i16)  [unwired: 6 in]
        n149 = call "GT Set Vel.vi"("error in (no error)"=w336, "vel"="vel", "profile"=w333, "cardNum"=w337) -> ("error out"=w335:errorcluster, "function return"=→"vel return":i16)  [unwired: 6 in]
        n150 = Decrement(x=w333) -> (x-1=w334:T5)
        n151 = Scale By Power Of 2(n=w334, x=ext 1.0) -> (x*2^n=w331:ext)
        n152 = call "GT Update.vi"("error in (no error)"=w335, "mask"=w331, "cardNum"=w337) -> ("function return"=→"updatereturn":i16)  [unwired: 7 in, 1 out]
      }
      event "插补运动": Mouse Down {
        w362 = i16 1 ("crd")
        w357 = i16 0 ("cardNum")
        # "插补文本(Crd_data)总共有500段数据，终点是50000pulse"
        n153 = event-data() -> ()  [unwired: 1 in, 8 out]
        n154 = call "GT Set Crd Prm.vi"("pCrdPrm"="pCrdPrm", "crd"=w362, "cardNum"=w357) -> ("error out"=w367:errorcluster, "function return"=→"setCrd return":i16)  [unwired: 7 in]
        n155 = call "GT Crd Clear.vi"("error in (no error)"=w367, "fifo"=i16 0, "crd"=w362, "cardNum"=w357) -> ("error out"=w365:errorcluster)  [unwired: 6 in, 1 out]
        n156 = case shown="True" "前瞻" {
          tunnel: w365 -> [w392 w402]
          tunnel: [w392 w401] -> w361
          tunnel: w357 -> [_ w400]
          tunnel: w362 -> [w391 w395]
          tunnel: [w391 w395] -> w359
          frame False {
          }
          frame True {
            n157 = call "GT Init Look Ahead.vi"("cardNum"=w400, "accMax"=1.0, "pLookAheadBuf"="pLookAheadBuf", "crd"=w395, "fifo"=i16 0, "T"=2.0, "error in (no error)"=w402, "n"=i16 200) -> ("function return"=→"lookahead":i16, "error out"=w401:errorcluster)  [unwired: 5 in, 1 out]
          }
        }
        n158 = Read from Text File(file (use dialog)="数据路径") -> (text=w351:string)  [unwired: 3 in, 3 out]
        n159 = for {
          N: 500 -> [_]
          tunnel: w359 -> [w371]
          tunnel: w357 -> [w370]
          tunnel: w351 -> [w375]
          tunnel: w361 -> [w383]
          tunnel: [w382] -> w358
          i -> [w373]
          n160 = Spreadsheet String To Array(format string="%d" ("格式字符串"), spreadsheet string=w375) -> (array=w374:dbl[][])  [unwired: 2 in]
          n161 = Index Array(array=w374, index (row)=w373) -> (element=w372:dbl[])  [unwired: 1 in]
          n162 = Index Array(array=w372, index=0 ("索引")) -> (element=w368:dbl)
          n163 = call "GT Ln XY.vi"("cardNum"=w370, "synVel"=10.0, "velEnd"=0.0, "crd"=w371, "x"=w368, "y"=w368, "error in (no error)"=w383, "synAcc"=1.0, "fifo"=i16 0) -> ("function return"=→"Lnxy return":i16, "error out"=w382:errorcluster)  [unwired: 5 in]
        }
        n164 = case shown="True" "前瞻" {
          tunnel: w357 -> [_ w390]
          tunnel: w359 -> [_ w389]
          tunnel: w358 -> [w384 w386]
          tunnel: [w384 w385] -> w353
          frame False {
          }
          frame True {
            n165 = call "GT Crd Data.vi"("fifo"=i16 0, "error in (no error)"=w386, "crd"=w389, "cardNum"=w390) -> ("error out"=w385:errorcluster, "function return"=→"crddata return":i16)  [unwired: 5 in, 1 out]
          }
        }
        n166 = call "GT Crd Start.vi"("error in (no error)"=w353, "option"=i16 0, "mask"=i16 1, "cardNum"=w357) -> ("function return"=→"CrdStart return":i16)  [unwired: 6 in, 1 out]
      }
      event "插补10000段": Mouse Down {
        w411 = 1
        w410 = 0
        n167 = event-data() -> ()  [unwired: 1 in, 8 out]
        n168 = local read "pCrdPrm"() -> (w416:T2)
        n169 = local read "前瞻"() -> (w413:bool)
        n170 = call "GT Set Crd Prm.vi"("pCrdPrm"=w416, "crd"=w411, "cardNum"=w410) -> ("error out"=w415:errorcluster)  [unwired: 7 in, 1 out]
        n171 = call "GT Crd Clear.vi"("error in (no error)"=w415, "fifo"=0, "crd"=w411, "cardNum"=w410) -> ("error out"=w412:errorcluster)  [unwired: 6 in, 1 out]
        n172 = case shown="True" w413 {
          tunnel: w412 -> [w436 w445]
          tunnel: w410 -> [_ w444]
          tunnel: w411 -> [_ w443]
          tunnel: [w436 w437] -> w409
          frame False {
          }
          frame True {
            n173 = local read "pLookAheadBuf"() -> (w439:T4)
            n174 = call "GT Init Look Ahead.vi"("cardNum"=w444, "accMax"=1.0, "pLookAheadBuf"=w439, "crd"=w443, "fifo"=0, "T"=2.0, "error in (no error)"=w445, "n"=200) -> ("error out"=w437:errorcluster)  [unwired: 5 in, 2 out]
          }
        }
        n175 = for {
          N: 4296 -> [_]
          tunnel: w409 -> [w435]
          tunnel: [w424] -> w407
          i -> [w432]
          n176 = Increment(x=w432) -> (x+1=w430:i32)
          n177 = Multiply(x=100, y=w430) -> (x*y=w429:i32)
          n178 = call "GT Ln XY.vi"("cardNum"=0, "synVel"=50.0, "velEnd"=0.0, "crd"=1, "x"=w429, "y"=w429, "error in (no error)"=w435, "synAcc"=1.0, "fifo"=0) -> ("error out"=w424:errorcluster)  [unwired: 5 in, 1 out]
        }
        n179 = call "GT Crd Start.vi"("error in (no error)"=w407, "option"=0, "mask"=1, "cardNum"=0) -> ("error out"=w403:errorcluster)  [unwired: 6 in, 1 out]
        n180 = while {
          tunnel: w403 -> [w418]
          stop <- FALSE stop-if-true
          w422 = 0
          n181 = call "GT Crd Space.vi"("fifo"=w422, "error in (no error)"=w418, "crd"=1, "cardNum"=w422) -> ("pSpace out"=w421:i32)  [unwired: 5 in, 2 out]
          n182 = Not Equal?(x=w421, y=0) -> (x != y?=w419:bool)
          n183 = case shown="True" w419 {
            frame False {
            }
            frame True {
            }
          }
        }
      }
      event "更新运动": Mouse Down {
        w448 = i16 0 ("cardNum")
        n184 = event-data() -> ()  [unwired: 1 in, 8 out]
        n185 = local read "轴号"() -> (w446:T5)
        n186 = local read "vel 2"() -> (w447:dbl)
        n187 = call "GT Set Vel.vi"("vel"=w447, "profile"=w446, "cardNum"=w448) -> ("error out"=w449:errorcluster)  [unwired: 7 in, 1 out]
        n188 = call "GT Update.vi"("error in (no error)"=w449, "mask"=w446, "cardNum"=w448) -> ("function return"=→"updatemotion return":i16)  [unwired: 7 in, 1 out]
      }
      event "闭环控制": Mouse Down {
        w455 = i16 0 ("cardNum")
        n189 = event-data() -> ()  [unwired: 1 in, 8 out]
        n190 = local read "轴号"() -> (w451:T5)
        n191 = call "GT Ctrl Mode.vi"("mode"=i16 0, "axis"=w451, "cardNum"=w455) -> ("error out"=w453:errorcluster, "function return"=w462:i16)  [unwired: 7 in]
        n192 = call "GT Clr Sts.vi"("error in (no error)"=w453, "count"=i16 4, "axis"=i16 1, "cardNum"=w455) -> ("error out"=w458:errorcluster, "function return"=w461:i16)  [unwired: 6 in]
        n193 = call "GT Get Pid.vi"("pPid"="闭环PID参数", "error in (no error)"=w458, "index"=i16 1, "control"=w451, "cardNum"=w455) -> ("error out"=w452:errorcluster, "function return"=w456:i16)  [unwired: 4 in, 1 out]
        n194 = call "GT Set Pid.vi"("pPid"="闭环PID参数", "error in (no error)"=w452, "index"=i16 1, "control"=w451, "cardNum"=w455) -> ("function return"=w460:i16)  [unwired: 4 in, 2 out]
        n195 = Build Array(w460, w456, w461, w462) -> (→"闭环返回值":i16[])
      }
      event "单次测试": Mouse Down {
        w467 = i16 0 ("cardNum")
        w485 = i16 0 ("cardNum")
        # "步骤：设置Follow运动、事件和任务、插补运动"
        n196 = event-data() -> ()  [unwired: 1 in, 8 out]
        n197 = local read "主轴"() -> (w473:i16)
        n198 = local read "pPrm 3"() -> (w477:cluster{"acc":dbl, "dec":dbl, "smooth":dbl})
        n199 = call "GT Prf Follow.vi"("dir"=i16 0, "profile"="从轴", "cardNum"=w485) -> ("error out"=w512:errorcluster)  [unwired: 7 in, 1 out]
        n200 = call "GT Follow Clear.vi"("error in (no error)"=w512, "fifo"=i16 0, "profile"="从轴", "cardNum"=w485) -> ("error out"=w510:errorcluster)  [unwired: 6 in, 1 out]
        n201 = local read "vel 2"() -> (w475:dbl)
        n202 = call "GT Set Follow Master.vi"("masterItem"=i16 0, "masterType"=i16 2, "error in (no error)"=w510, "masterIndex"="主轴", "profile"="从轴", "cardNum"=w485) -> ("error out"=w507:errorcluster)  [unwired: 4 in, 1 out]
        n203 = Decrement(x=w473) -> (x-1=w472:i16)
        n204 = Scale By Power Of 2(n=w472, x=ext 1.0) -> (x*2^n=w470:ext)
        n205 = call "GT Follow Data.vi"("fifo"=i16 0, "type"=i16 0, "slaveSegment"=5000.0, "error in (no error)"=w507, "masterSegment"=20000, "profile"="从轴", "cardNum"=w485) -> ("error out"=w502:errorcluster)  [unwired: 3 in, 1 out]
        n206 = call "GT Follow Data.vi"("fifo"=i16 0, "type"=i16 1, "slaveSegment"=30000.0, "error in (no error)"=w502, "masterSegment"=40000, "profile"="从轴", "cardNum"=w485) -> ("error out"=w501:errorcluster)  [unwired: 3 in, 1 out]
        n207 = call "GT Follow Data.vi"("fifo"=i16 0, "type"=i16 0, "slaveSegment"=0.0, "error in (no error)"=w501, "masterSegment"=80000, "profile"="从轴", "cardNum"=w485) -> ("error out"=w491:errorcluster)  [unwired: 3 in, 1 out]
        n208 = call "GT Set Follow Loop.vi"("error in (no error)"=w491, "loop"=1, "profile"="从轴", "cardNum"=w485) -> ("error out"=w489:errorcluster)  [unwired: 6 in, 1 out]
        n209 = call "GT Set Follow Event.vi"("pos"=30000, "masterDir"=i16 1, "error in (no error)"=w489, "event"=i16 2, "profile"="从轴", "cardNum"=w485) -> ("error out"=w486:errorcluster)  [unwired: 4 in, 1 out]
        n210 = Decrement(x="从轴") -> (x-1=w484:i16)
        n211 = Scale By Power Of 2(n=w484, x=ext 1.0) -> (x*2^n=w481:ext)
        n212 = call "GT Follow Start.vi"("error in (no error)"=w486, "option"=0, "mask"=w481, "cardNum"=w485) -> ("error out"=w479:errorcluster)  [unwired: 6 in, 1 out]
        n213 = call "GT Prf Jog.vi"("error in (no error)"=w479, "profile"=w473, "cardNum"=w467) -> ("error out"=w478:errorcluster)  [unwired: 7 in, 1 out]
        n214 = call "GT Get Jog Prm.vi"("error in (no error)"=w478, "pPrm"=w477, "profile"=w473, "cardNum"=w467) -> ("error out"=w476:errorcluster)  [unwired: 5 in, 2 out]
        n215 = call "GT Set Jog Prm.vi"("error in (no error)"=w476, "pPrm"=w477, "profile"=w473, "cardNum"=w467) -> ("error out"=w474:errorcluster)  [unwired: 5 in, 2 out]
        n216 = call "GT Set Vel.vi"("error in (no error)"=w474, "vel"=w475, "profile"=w473, "cardNum"=w467) -> ("error out"=w469:errorcluster)  [unwired: 6 in, 1 out]
        n217 = call "GT Update.vi"("error in (no error)"=w469, "mask"=w470, "cardNum"=w467) -> ("error out"=w468:errorcluster)  [unwired: 7 in, 1 out]
        n218 = disable-structure shown="禁用" {
          disable-tunnel: w468 -> [w536 _]
          disable-tunnel: w467 -> [w527 _]
          frame Disabled {
            n219 = call "GT Add Task.vi"("error in (no error)"=w536, "pTaskData"="pTaskData", "taskType"=i16 16388, "cardNum"=w527) -> ("error out"=w534:errorcluster, "pTaskIndex out"=w532:i16)  [unwired: 4 in, 2 out]
            n220 = call "GT Add Event.vi"("error in (no error)"=w534, "pEvent"="pEvent", "cardNum"=w527) -> ("error out"=w531:errorcluster, "pEventIndex out"=w530:i16)  [unwired: 5 in, 2 out]
            n221 = call "GT Add Event Task Link.vi"("error in (no error)"=w531, "taskIndex"=w532, "eventIndex"=w530, "cardNum"=w527) -> ("error out"=w528:errorcluster)  [unwired: 5 in, 2 out]
            n222 = local read "pCrdPrm"() -> (w524:T2)
            n223 = call "GT Event On.vi"("error in (no error)"=w528, "count"=i16 1, "eventIndex"=w530, "cardNum"=w527) -> ("error out"=w525:errorcluster)  [unwired: 6 in, 1 out]
            n224 = call "GT Set Crd Prm.vi"("error in (no error)"=w525, "pCrdPrm"=w524, "crd"=i16 1, "cardNum"=w527) -> ("error out"=w523:errorcluster)  [unwired: 6 in, 1 out]
            n225 = call "GT Ln XY.vi"("cardNum"=i16 0, "synVel"=3.0, "velEnd"=0.0, "crd"=i16 1, "x"=20000, "y"=20000, "error in (no error)"=w523, "synAcc"=1.0, "fifo"=i16 0) -> ()  [unwired: 5 in, 2 out]
          }
          frame Enabled {
          }
        }
      }
      event Application Instance Close {
        w540 = i16 0 ("cardNum")
        n226 = event-data() -> ()  [unwired: 1 in, 4 out]
        n227 = call "GT Reset.vi"("cardNum"=w540) -> ("error out"=w539:errorcluster)  [unwired: 9 in, 1 out]
        n228 = call "GT Close Ext Mdl.vi"("error in (no error)"=w539, "cardNum"=w540) -> ("error out"=w538:errorcluster)  [unwired: 8 in, 1 out]
        n229 = call "GT Close.vi"("error in (no error)"=w538, "cardNum"=w540) -> ()  [unwired: 8 in, 2 out]
      }
      event "关伺服": Mouse Down {
        w545 = i16 0 ("axis")
        # "关伺服"
        n230 = event-data() -> ()  [unwired: 1 in, 8 out]
        n231 = call "GT Axis Off.vi"("axis"=i16 1, "cardNum"=w545) -> ("error out"=w546:errorcluster, "function return"=→"Axisoff return":i16)  [unwired: 8 in]
        n232 = call "GT Axis Off.vi"("error in (no error)"=w546, "axis"=i16 2, "cardNum"=w545) -> ("error out"=w544:errorcluster)  [unwired: 7 in, 1 out]
        n233 = call "GT Axis Off.vi"("error in (no error)"=w544, "axis"=i16 3, "cardNum"=w545) -> ("error out"=w543:errorcluster)  [unwired: 7 in, 1 out]
        n234 = call "GT Axis Off.vi"("error in (no error)"=w543, "axis"=i16 4, "cardNum"=w545) -> ()  [unwired: 7 in, 2 out]
      }
      event "清零": Mouse Down {
        n235 = event-data() -> ()  [unwired: 1 in, 8 out]
        n236 = call "GT Zero Pos.vi"("count"=i16 8, "axis"=i16 1, "cardNum"=i16 0) -> ("function return"=→"zero return":i16)  [unwired: 7 in, 1 out]
      }
      event "初始化扩展模块": Mouse Down {
        w557 = 0
        n237 = event-data() -> ()  [unwired: 1 in, 8 out]
        n238 = call "GT Open Ext Mdl.vi"("pDllName"="pDllName", "cardNum"=w557) -> ("function return"=→"function return":i16)  [unwired: 7 in, 2 out]
        n239 = Path To String(path="路径 2") -> (string=w555:string)
        n240 = call "GT Load Ext Config.vi"("pFileName"=w555, "cardNum"=w557) -> ("function return"=→"function return 2":i16)  [unwired: 7 in, 2 out]
      }
      event "SetDo": Mouse Down {
        n241 = event-data() -> ()  [unwired: 1 in, 8 out]
        n242 = call "GT Set Ext Io Bit.vi"("value"="value", "index"="index", "mdl"="mdl", "cardNum"=0) -> ("function return"=→"function return 3":i16)  [unwired: 6 in, 1 out]
      }
      event "位置比较": Mouse Down {
        w568 = 0
        w578 = 0
        n243 = event-data() -> ()  [unwired: 1 in, 8 out]
        n244 = disable-structure shown="禁用" {
          disable-tunnel: "pBuf" -> [w603 _]
          frame Disabled {
            w596 = 0
            n245 = call "GT 2D Compare Clear.vi"("chn"=1, "cardNum"=w596) -> ("error out"=w601:errorcluster, "function return"=w590:i16)  [unwired: 8 in]
            n246 = call "GT 2D Compare Mode.vi"("error in (no error)"=w601, "mode"=0, "chn"=1, "cardNum"=w596) -> ("error out"=w595:errorcluster, "function return"=w589:i16)  [unwired: 6 in]
            n247 = call "GT 2D Compare Set Prm.vi"("error in (no error)"=w595, "pPrm"="pPrm 4", "chn"=1, "cardNum"=w596) -> ("error out"=w592:errorcluster, "function return"=w588:i16)  [unwired: 5 in, 1 out]
            n248 = call "GT 2D Compare Data.vi"("fifo"=0, "pBuf"=w603, "error in (no error)"=w592, "count"=6, "chn"=1, "cardNum"=w596) -> ("function return"=w587:i16)  [unwired: 3 in, 2 out]
            n249 = Build Array(w590, w589, w588, w587) -> (→"比较2return":i16[])
          }
          frame Enabled {
          }
        }
        n250 = call "GT 2D Compare Clear Data.vi"("chn"=w568, "cardNum"=w568) -> ("error out"=w566:errorcluster, "function return"=w567:i16)  [unwired: 8 in]
        n251 = call "GT 2D Compare Clear.vi"("error in (no error)"=w566, "chn"=0, "cardNum"=w568) -> ("error out"=w565:errorcluster, "function return"=w574:i16)  [unwired: 7 in]
        n252 = call "GT 2D Compare Mode.vi"("error in (no error)"=w565, "mode"=0, "chn"=0, "cardNum"=w578) -> ("error out"=w576:errorcluster, "function return"=w573:i16)  [unwired: 6 in]
        n253 = call "GT 2D Compare Set Prm.vi"("error in (no error)"=w576, "pPrm"="pPrm 2", "chn"=0, "cardNum"=w578) -> ("error out"=w579:errorcluster, "function return"=w572:i16)  [unwired: 5 in, 1 out]
        n254 = call "GT 2D Compare Data.vi"("fifo"=0, "pBuf"="pBuf", "error in (no error)"=w579, "count"=6, "chn"=0, "cardNum"=w578) -> ("function return"=w571:i16)  [unwired: 3 in, 2 out]
        n255 = Build Array(w574, w573, w572, w571, w567) -> (→"比较1return":i16[])
      }
      event "启动位置比较": Mouse Down {
        n256 = event-data() -> ()  [unwired: 1 in, 8 out]
        n257 = disable-structure shown="禁用" {
          disable-tunnel: [w611 _] -> w605
          frame Disabled {
            n258 = call "GT 2D Compare Start.vi"("chn"=1, "cardNum"=0) -> ("function return"=w611:i16)  [unwired: 8 in, 1 out]
          }
          frame Enabled {
          }
        }
        n259 = call "GT 2D Compare Start.vi"("chn"=0, "cardNum"=0) -> ("function return"=w606:i16)  [unwired: 8 in, 1 out]
        n260 = Build Array(w606, w605) -> (→"comparestart return":i16[])
      }
      event "停止位置比较": Mouse Down {
        n261 = event-data() -> ()  [unwired: 1 in, 8 out]
        n262 = call "GT 2D Compare Stop.vi"("chn"=0, "cardNum"=0) -> ("error out"=w612:errorcluster, "function return"=w615:i16)  [unwired: 8 in]
        n263 = disable-structure shown="禁用" {
          disable-tunnel: [w621 _] -> w614
          disable-tunnel: w612 -> [w620 _]
          frame Disabled {
            n264 = call "GT 2D Compare Stop.vi"("error in (no error)"=w620, "chn"=1, "cardNum"=0) -> ("function return"=w621:i16)  [unwired: 7 in, 1 out]
          }
          frame Enabled {
          }
        }
        n265 = Build Array(w615, w614) -> (→"comparestop return":i16[])
      }
      event "三轴直线插补": Mouse Down {
        w632 = 50000
        w634 = 0
        w635 = 1
        w636 = 0.0
        w637 = 5.0
        w640 = 10000
        w633 = 1
        w631 = 0
        n266 = event-data() -> ()  [unwired: 1 in, 8 out]
        n267 = call "GT Set Crd Prm.vi"("pCrdPrm"="pCrdPrm 2", "crd"=w633, "cardNum"=w631) -> ("error out"=w641:errorcluster, "function return"=w627:i16)  [unwired: 7 in]
        n268 = call "GT Crd Clear.vi"("error in (no error)"=w641, "fifo"=0, "crd"=w633, "cardNum"=w631) -> ("error out"=w639:errorcluster, "function return"=w626:i16)  [unwired: 6 in]
        n269 = call "GT Ln XYZ.vi"("cardNum"=w631, "z"=w640, "synAcc"=w635, "fifo"=w634, "crd"=w633, "x"=w640, "y"=w640, "error in (no error)"=w639, "synVel"=w637, "velEnd"=w636) -> ("function return"=w625:i16, "error out"=w638:errorcluster)  [unwired: 4 in]
        n270 = call "GT Ln XYZ.vi"("cardNum"=w631, "z"=w632, "synAcc"=w635, "fifo"=w634, "crd"=w633, "x"=w632, "y"=w632, "error in (no error)"=w638, "synVel"=w637, "velEnd"=w636) -> ("function return"=w624:i16, "error out"=w630:errorcluster)  [unwired: 4 in]
        n271 = call "GT Crd Start.vi"("error in (no error)"=w630, "option"=i16 0, "mask"=1, "cardNum"=w631) -> ("function return"=w623:i16)  [unwired: 6 in, 1 out]
        n272 = Build Array(w627, w626, w625, w624, w623) -> (→"添加的数组":i16[])
      }
      event "一维位置比较": Mouse Down {
        n273 = event-data() -> ()  [unwired: 1 in, 8 out]
        n274 = call "GT Set Capture Mode.vi"("mode"=6, "encoder"=1, "cardNum"=0) -> ("error out"=w645:errorcluster, "function return"=→"function return 7":i16)  [unwired: 7 in]
        n275 = call "GT Compare Data.vi"("cardNum"=0, "encoder"=1, "source"=0, "pulseType"=0, "startLevel"=0, "time"=10000, "pBuf1"="pBuf1", "error in (no error)"=w645, "count1"=1) -> ("function return"=→"function return 6":i16)  [unwired: 16 in, 2 out]
      }
      event "关卡": Mouse Down {
        n276 = event-data() -> ()  [unwired: 1 in, 8 out]
        n277 = call "GT Close.vi"("cardNum"=0) -> ("function return"=→"close return":i16)  [unwired: 9 in, 1 out]
      }
    }
    n278 = Wait (ms)(milliseconds to wait=u32 500 ("等待时间（毫秒）")) -> ()  [unwired: 1 out]
  }
  n279 = while {
    stop <- FALSE stop-if-true
    n280 = case shown="True" "打开home捕获" {
      frame False {
      }
      frame True {
        n281 = while {
          i -> [w664]
          stop <- FALSE stop-if-true
          n282 = flat-sequence {
            tunnel: [w670] -> w663
            tunnel: w664 -> [_]
            tunnel: w663 -> [w679]
            frame #0 {
              n283 = call "GT Set Capture Mode.vi"("mode"=i16 1, "encoder"=i16 1, "cardNum"=i16 0) -> ()  [unwired: 7 in, 2 out]
            }
            frame #1 {
              n284 = while {
                tunnel: [w672] -> w670
                stop <- w673 continue-if-true
                n285 = call "GT Get Capture Status.vi"("cardNum"=i16 0, "count"=i16 1, "encoder"=i16 1) -> ("pStatus out"=w674:i16, "pValue out"=w672:i32)  [unwired: 8 in, 3 out]
                n286 = Equal To 0?(x=w674) -> (x = 0?=w673:bool)
                n287 = Wait (ms)(milliseconds to wait=u32 100 ("等待时间（毫秒）")) -> ()  [unwired: 1 out]
              }
            }
            frame #2 {
              n288 = local read "捕获数组"() -> (w681:i32[])
              n289 = local read "捕获次数"() -> (w678:i32)
              n290 = Replace Array Subset(array=w681, new element=w679, index=w678) -> (w680:i32[])
              n291 = local write "捕获数组"(w680) -> ()
              "pValue out" <- w679
            }
            frame #3 {
              n292 = local read "捕获次数"() -> (w683:i32)
              n293 = Increment(x=w683) -> (x+1=w682:i32)
              n294 = local write "捕获次数"(w682) -> ()
            }
          }
          n295 = Wait (ms)(milliseconds to wait=u32 200 ("等待时间（毫秒）")) -> ()  [unwired: 1 out]
        }
      }
    }
    n296 = Wait (ms)(milliseconds to wait=u32 200 ("等待时间（毫秒）")) -> ()  [unwired: 1 out]
  }
  n297 = while {
    stop <- FALSE stop-if-true
    # "停止所有轴运动"
    n298 = Wait (ms)(milliseconds to wait=u32 200 ("等待时间（毫秒）")) -> ()  [unwired: 1 out]
    n299 = case shown="True" "停止" {
      frame False {
      }
      frame True {
        n300 = call "GT Stop.vi"("option"=0, "mask"=255, "cardNum"=0 ("mask")) -> ("function return"=→"stopreturn":i16)  [unwired: 7 in, 1 out]
      }
    }
  }
  "捕获数组" <- i32[] [0, 0, 0, 0, 0, 0, 0, 0, 0, 0, 0, 0, 0, 0, 0, 0, 0, 0, 0, 0, 0, 0, 0, 0, 0, 0, 0, 0, 0, 0, 0, 0, 0, 0, 0, 0, 0, 0, 0, 0, 0, 0, 0, 0, 0, 0, 0, 0, 0, 0, 0, 0, 0, 0, 0, 0, 0, 0, 0, 0, 0, 0, 0, 0, 0, 0, 0, 0, 0, 0, 0, 0, 0, 0, 0, 0, 0, 0, 0, 0, 0, 0, 0, 0, 0, 0, 0, 0, 0, 0, 0, 0, 0, 0, 0, 0, 0, 0, 0, 0, 0] ("捕获数组 2")
  "捕获次数" <- 0 ("捕获次数")
